vi "List Group Objects.vi"(6 "error in (no error)":errorcluster, 7 "Object Types (any)":T1[](array[typedef]) items=["H5G_UNKNOWN"=-1, "H5G_GROUP"=0, "H5G_DATASET"=1, "H5G_TYPE"=2, "H5G_LINK"=3, "H5G_UDLINK"=4], 8 "pattern":string, 9 "HDF5 Loc Ref":T2) -> (0 "error out":errorcluster, 1 "Obect Types":T1[](array[typedef]) items=["H5G_UNKNOWN"=-1, "H5G_GROUP"=0, "H5G_DATASET"=1, "H5G_TYPE"=2, "H5G_LINK"=3, "H5G_UDLINK"=4], 2 "Object Names":string[](array[string]), 3 "HDF5 Loc Ref out":T2)   [LabVIEW 2017]
doc: "Lists some or all of the objects at a given location"
uses:
  <vilib>/UPVI/lvhdf5/group.llb/H5G_obj_t.ctl
  <vilib>/UPVI/lvhdf5/library.llb/HDF5 Ref.ctl
  <userlib>/_OpenG.lib/array/array.llb/Conditional Auto-Indexing Tunnel (I32)__ogtk.vi
  <userlib>/_OpenG.lib/array/array.llb/Conditional Auto-Indexing Tunnel (String)__ogtk.vi
panel:
  # "LVHDF5 Toolkit\nCopyright (c) 2005-2013 by Jason D. Sommerville\nCopyright (c) 2014 by UPVI, LLC.\n\nThis use and distribution of this file is governed by the terms found in \nLICENSE.txt distributed with this toolkit and installed at\n <user.lib>\\_lvhdf5\\LICENSE.txt"
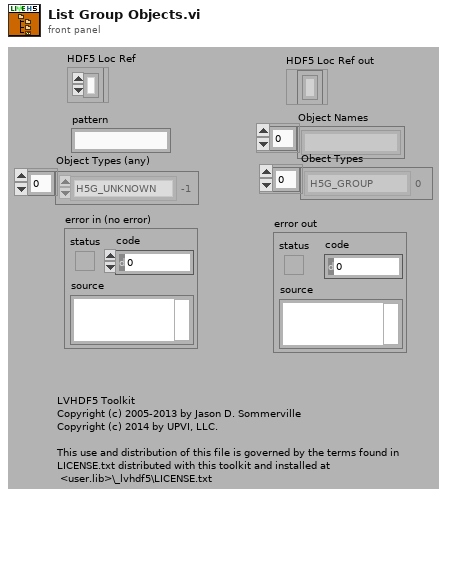
[diagram p1: front panel]
types:
  T1 = typedef "H5G_obj_t.ctl" = i32
  T2 = typedef "HDF5 Ref.ctl" = refnum<k1>
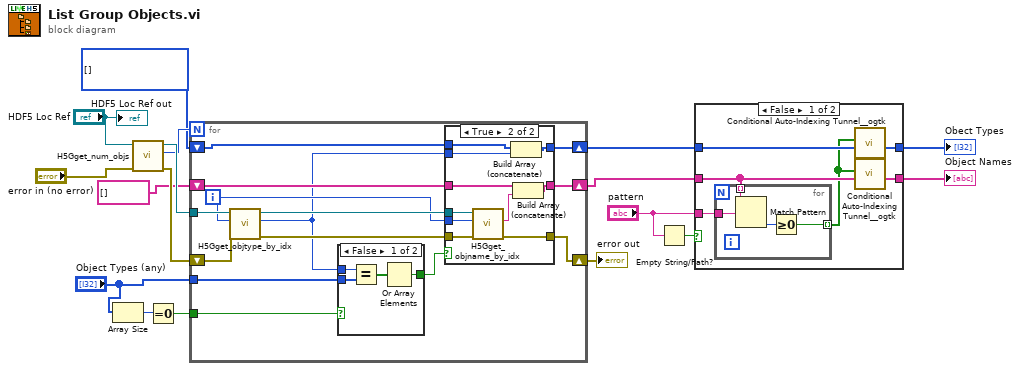
[diagram p0: block diagram]
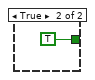
[diagram p4: hidden frame]
diagram:
  w10 = T1[] [] items=["H5G_UNKNOWN"=-1, "H5G_LINK"=0, "H5G_GROUP"=1, "H5G_DATASET"=2, "H5G_TYPE"=3]
  n1 = Array Size(array="Object Types (any)") -> (size(s)=w2:i32)
  n2 = call <vilib>:"H5Gget_num_objs.vi"("error in (no error)"="error in (no error)", "HDF5 Ref"="HDF5 Loc Ref") -> ("error out"=w15:errorcluster, "Count"=w14:u64, "HDF5 Ref out"=w16:T2)  [unwired: 5 in]
  n3 = Equal To 0?(x=w2) -> (x = 0?=w1:bool)
  n4 = for {
    N: w14 -> [_]
    shift-right: [w26] -> w17
    shift-left: w15 -> [w31]
    tunnel: "Object Types (any)" -> [w30]
    tunnel: w16 -> [w29]
    shift-right: [w24] -> w5
    shift-left: string[] [] -> [w23]
    shift-right: [w20] -> w7
    shift-left: w10 -> [w19]
    tunnel: w1 -> [w18]
    i -> [w22]
    n5 = call <vilib>:"H5Gget_objtype_by_idx.vi"("error in (no error)"=w31, "Index"=w22, "HDF5 Ref"=w29) -> ("error out"=w27:errorcluster, "Object Type"=w21:T1, "HDF5 Ref out"=w25:T2)  [unwired: 4 in]
    n6 = case shown="False" w18 {
      tunnel: w21 -> [w48 _]
      tunnel: w30 -> [w47 _]
      tunnel: [w45 TRUE] -> w28
      frame False {
        n7 = Equal?(x=w48, y=w47) -> (x = y?=w46:bool[])
        n8 = Or Array Elements(Boolean array=w46) -> (logical OR=w45:bool)
      }
      frame True {
      }
    }
    n9 = case shown="True" w28 {
      tunnel: w27 -> [w33 w44]
      tunnel: [w33 w43] -> w26
      tunnel: w25 -> [_ w42]
      tunnel: [w34 w40] -> w24
      tunnel: w23 -> [w34 w39]
      tunnel: w22 -> [_ w38]
      tunnel: w21 -> [_ w37]
      tunnel: [w32 w36] -> w20
      tunnel: w19 -> [w32 w35]
      frame False {
      }
      frame True {
        n10 = call <vilib>:"H5Gget_objname_by_idx.vi"("error in (no error)"=w44, "Index"=w38, "HDF5 Ref"=w42) -> ("error out"=w43:errorcluster, "Name"=w41:string)  [unwired: 4 in, 1 out]
        n11 = Build Array (concatenate)(w35, w37) -> (w36:T1[])
        n12 = Build Array (concatenate)(w39, w41) -> (w40:string[])
      }
    }
  }
  "error out" <- w17
  n13 = Empty String/Path?(string/path="pattern") -> (empty?=w9:bool)
  n14 = case shown="False" w9 {
    tunnel: "pattern" -> [w55 _]
    tunnel: w5 -> [w54 w60]
    tunnel: w7 -> [w53 w61]
    tunnel: [w51 w61] -> w6
    tunnel: [w50 w60] -> w4
    frame False {
      n15 = for {
        tunnel: w55 -> [w59]
        tunnel: [w57] -> w52 mode=indexing
        tunnel: w54 -> [w56] mode=indexing
        n16 = Match Pattern(string=w56, regular expression=w59) -> (offset past match=w58:i32)  [unwired: 1 in, 3 out]
        n17 = Greater Or Equal To 0?(x=w58) -> (x >= 0?=w57:bool)
      }
      n18 = call-poly <userlib>:"Conditional Auto-Indexing Tunnel__ogtk.vi"("Array in"=w53, "Elements to keep"=w52) -> ("Filtered Array out"=w51:i32[])  [unwired: 5 in]
      n19 = call-poly <userlib>:"Conditional Auto-Indexing Tunnel__ogtk.vi"("Array in"=w54, "Elements to keep"=w52) -> ("Filtered Array out"=w50:string[])  [unwired: 5 in]
    }
    frame True {
    }
  }
  "Object Names" <- w4
  "Obect Types" <- w6
  "HDF5 Loc Ref out" <- "HDF5 Loc Ref"
